vi "WaferMap Example (LabVIEW2014).vi"() -> ()   [LabVIEW 2014]
doc: "This example detects and responds to a service request (SRQ) event. It shows a generic method to generate and handle an SRQ event. But each instrument that supports SRQ event assertion will use a different set of commands than what is shown in this example. You will need to refer to the programmer reference manual for your particular instrument to determine the correct set of commands."
panel:
  out "Home":string
  out "Grid":string
  out "flat":string
  out "die info":string
  out "WaferSize":string
  out "Machine":string
  in  "VISA GPIB Resource":refnum<visa-resource-name>="GPIB0::13::INSTR"
  # "SENTIO Remote Control Example - Wafer Map Setup"
  # "Step 5: Setup the Home Die"
  # "Query Machine"
  # "Step 1: StepUpWaferSize"
  # "Step 4: Setup the Origin"
  # "Step 2: StepUpDieSize"
  # "Step 3: SetUp Flat"
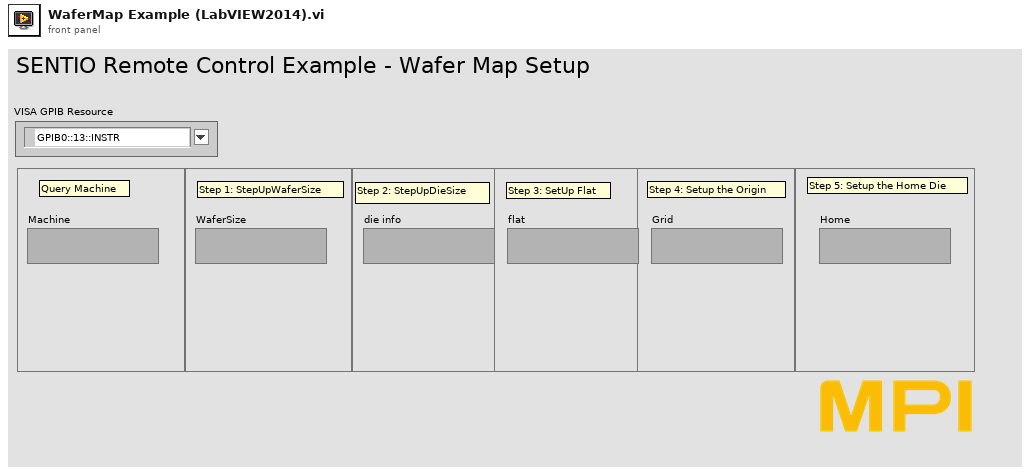
[diagram p1: front panel]
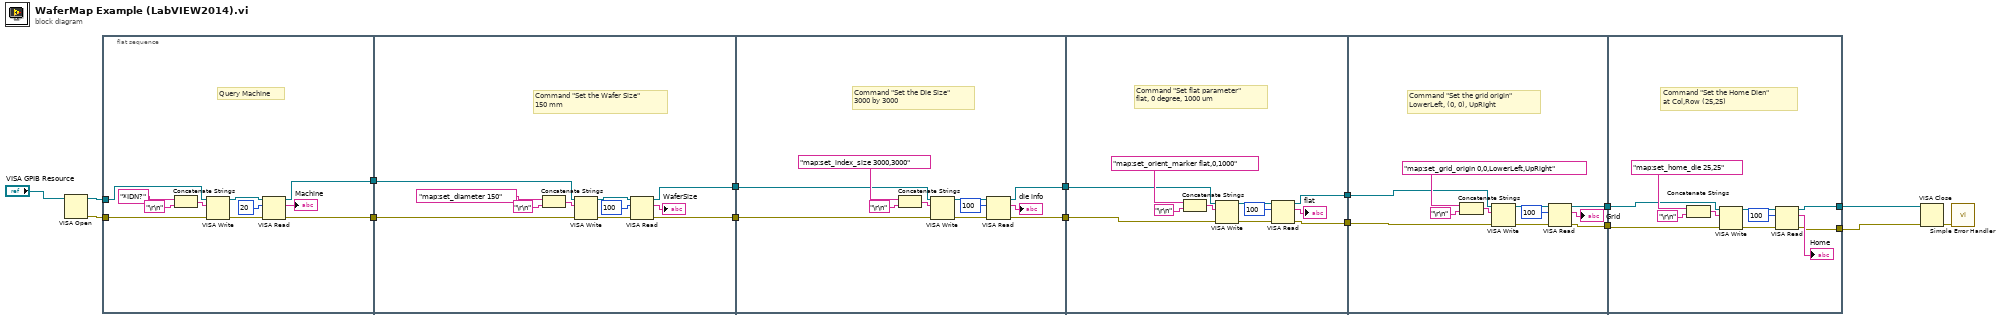
[diagram p0: block diagram]
diagram:
  n1 = VISA Open(VISA resource name="VISA GPIB Resource") -> (VISA resource name=w15:refnum<visa-resource-name>, error out=w14:errorcluster)  [unwired: 1 in, 3 out]
  n2 = flat-sequence {
    tunnel: w15 -> [w27]
    tunnel: w14 -> [w26]
    tunnel: [w21] -> w13
    tunnel: [w20] -> w12
    tunnel: [w29] -> w11
    tunnel: [w28] -> w10
    tunnel: w13 -> [w35]
    tunnel: w12 -> [w34]
    tunnel: w11 -> [w44]
    tunnel: w10 -> [w43]
    tunnel: [w42] -> w9
    tunnel: [w41] -> w8
    tunnel: w9 -> [w53]
    tunnel: w8 -> [w52]
    tunnel: [w51] -> w6
    tunnel: [w50] -> w5
    tunnel: w6 -> [w64]
    tunnel: w5 -> [w63]
    tunnel: [w62] -> w4
    tunnel: [w61] -> w3
    tunnel: w4 -> [w75]
    tunnel: w3 -> [w74]
    tunnel: [w73] -> w2
    tunnel: [w72] -> w1
    frame #0 {
      # "Query Machine"
      n3 = Concatenate Strings("*IDN?" ("write buffer"), "\r\n") -> (w17:string)
      n4 = VISA Write(VISA resource name=w27, write buffer=w17, error in (no error)=w26) -> (VISA resource name out=w23:refnum<visa-resource-name>, error out=w22:errorcluster)  [unwired: 1 out]
      n5 = VISA Read(VISA resource name=w23, byte count=u32 20, error in (no error)=w22) -> (VISA resource name out=w21:refnum<visa-resource-name>, read buffer=→"Machine":string, error out=w20:errorcluster)  [unwired: 1 out]
    }
    frame #1 {
      # "Command \"Set the Wafer Size\"\n150 mm"
      n6 = Concatenate Strings("map:set_diameter 150" ("Command"), "\r\n") -> (w38:string)
      n7 = VISA Write(VISA resource name=w35, write buffer=w38, error in (no error)=w34) -> (VISA resource name out=w31:refnum<visa-resource-name>, error out=w30:errorcluster)  [unwired: 1 out]
      n8 = VISA Read(VISA resource name=w31, byte count=u32 100, error in (no error)=w30) -> (VISA resource name out=w29:refnum<visa-resource-name>, read buffer=→"WaferSize":string, error out=w28:errorcluster)  [unwired: 1 out]
    }
    frame #2 {
      # "Command \"Set the Die Size\"\n3000 by 3000"
      n9 = Concatenate Strings("map:set_index_size 3000,3000" ("Command"), "\r\n") -> (w45:string)
      n10 = VISA Write(VISA resource name=w44, write buffer=w45, error in (no error)=w43) -> (VISA resource name out=w40:refnum<visa-resource-name>, error out=w49:errorcluster)  [unwired: 1 out]
      n11 = VISA Read(VISA resource name=w40, byte count=u32 100, error in (no error)=w49) -> (VISA resource name out=w42:refnum<visa-resource-name>, read buffer=→"die info":string, error out=w41:errorcluster)  [unwired: 1 out]
    }
    frame #3 {
      # "Command \"Set flat parameter\"\nflat, 0 degree, 1000 um"
      n12 = Concatenate Strings("map:set_orient_marker flat,0,1000" ("Command"), "\r\n") -> (w58:string)
      n13 = VISA Write(VISA resource name=w53, write buffer=w58, error in (no error)=w52) -> (VISA resource name out=w59:refnum<visa-resource-name>, error out=w54:errorcluster)  [unwired: 1 out]
      n14 = VISA Read(VISA resource name=w59, byte count=u32 100, error in (no error)=w54) -> (VISA resource name out=w51:refnum<visa-resource-name>, read buffer=→"flat":string, error out=w50:errorcluster)  [unwired: 1 out]
    }
    frame #4 {
      # "Command \"Set the grid origin\"\nLowerLeft, (0, 0), UpRight"
      n15 = Concatenate Strings("map:set_grid_origin 0,0,LowerLeft,UpRight" ("Command"), "\r\n") -> (w67:string)
      n16 = VISA Write(VISA resource name=w64, write buffer=w67, error in (no error)=w63) -> (VISA resource name out=w66:refnum<visa-resource-name>, error out=w71:errorcluster)  [unwired: 1 out]
      n17 = VISA Read(VISA resource name=w66, byte count=u32 100, error in (no error)=w71) -> (VISA resource name out=w62:refnum<visa-resource-name>, read buffer=→"Grid":string, error out=w61:errorcluster)  [unwired: 1 out]
    }
    frame #5 {
      # "Command \"Set the Home Dien\"\nat Col,Row (25,25)"
      n18 = Concatenate Strings("map:set_home_die 25,25" ("Command"), "\r\n") -> (w80:string)
      n19 = VISA Write(VISA resource name=w75, write buffer=w80, error in (no error)=w74) -> (VISA resource name out=w81:refnum<visa-resource-name>, error out=w76:errorcluster)  [unwired: 1 out]
      n20 = VISA Read(VISA resource name=w81, byte count=u32 100, error in (no error)=w76) -> (VISA resource name out=w73:refnum<visa-resource-name>, read buffer=→"Home":string, error out=w72:errorcluster)  [unwired: 1 out]
    }
  }
  n21 = VISA Close(VISA resource name=w2, error in (no error)=w1) -> (error out=w7:errorcluster)
  n22 = call <vilib>:"Simple Error Handler.vi"("error in (no error)"=w7) -> ()  [unwired: 1 in, 8 out]
